vi "SDCP SMF Receiver and Transmitter - Notifiers and Queues FGV.vi"(2 "error in (no error)":errorcluster, 3 "Command":enum16{"Initialize", "Read", "Deinitialize"}(ring)) -> (0 "error out":errorcluster, 1 "Output":T1)   [LabVIEW 2020]
uses:
  Typedefs/SDCP SMF Receiver and Transmitter - Notifier and Queues.ctl
  Typedefs/SDCP SMF logger - SMF with timestamp.ctl
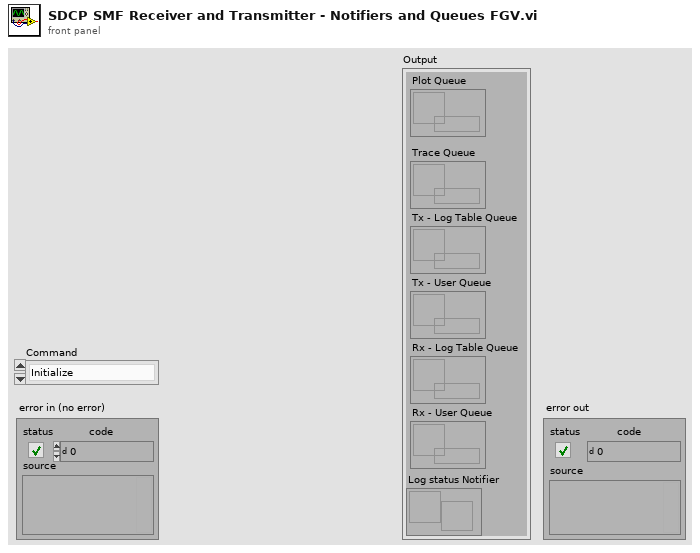
[diagram p1: front panel]
types:
  T1 = typedef "SDCP SMF Receiver and Transmitter - Notifier and Queues.ctl" = cluster{"Trace Queue":refnum<queue>, "Tx - Log Table Queue":refnum<queue>, "Tx - User Queue":refnum<queue>, "Rx - Log Table Queue":refnum<queue>, "Rx - User Queue":refnum<queue>, "Log status Notifier":refnum<notifier>, "Plot Queue":refnum<queue>}
  T2 = typedef "SDCP SMF logger - SMF with timestamp.ctl" = cluster{"Bytes":u8[], "Checksum":bool, "Time (ms)":u32, "Tx/Rx":string}
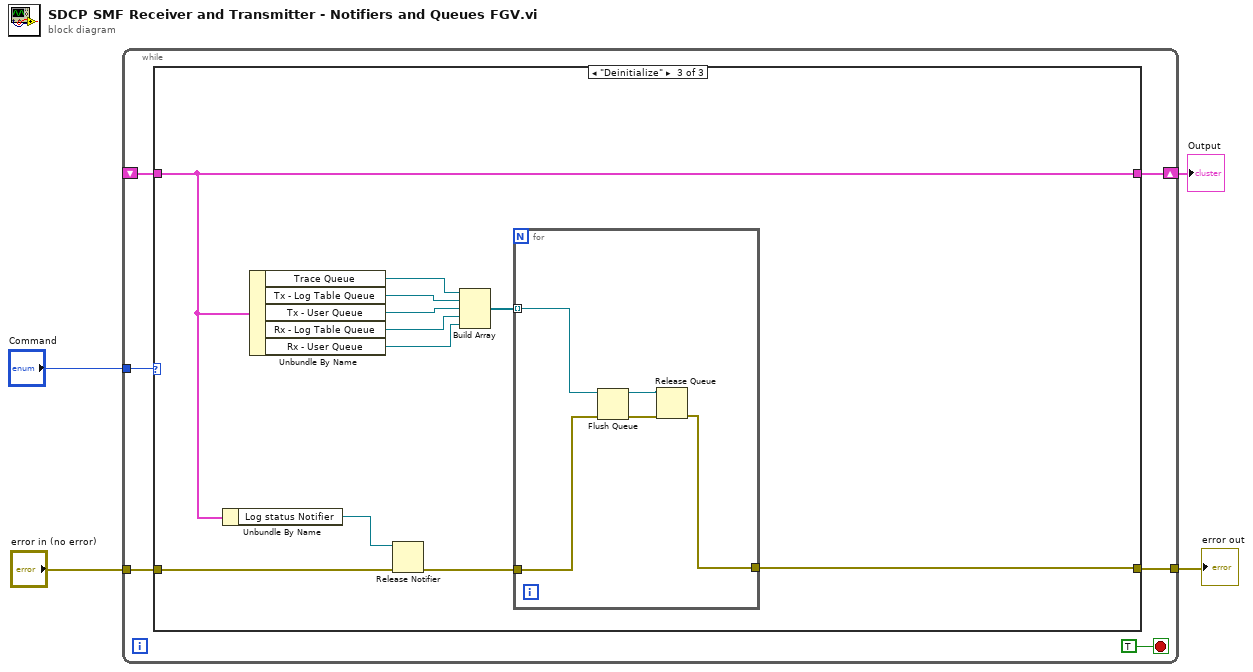
[diagram p0: block diagram]
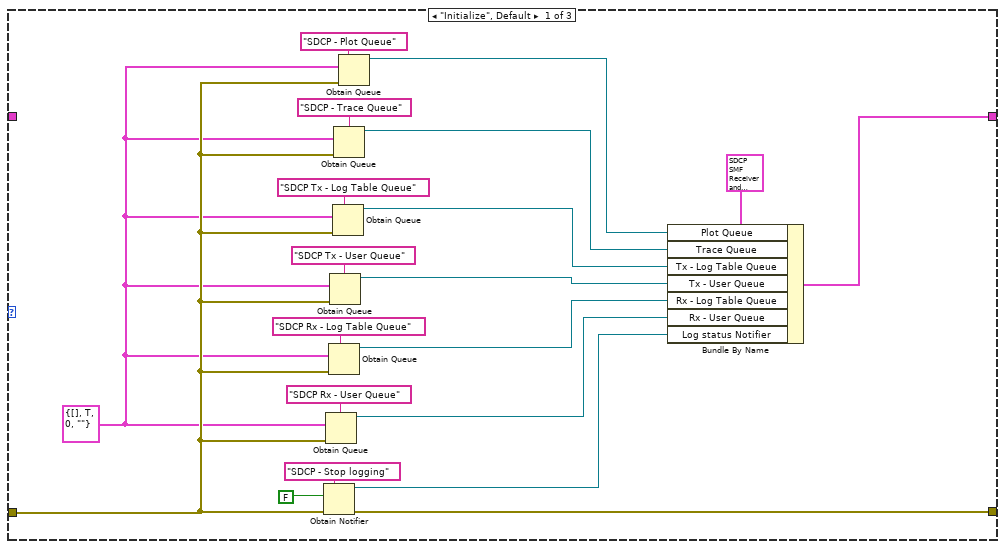
[diagram p2: hidden frame]
diagram:
  n1 = while {
    tunnel: "error in (no error)" -> [w8]
    tunnel: "Command" -> [w9]
    shift-right: [w7] -> w1
    shift-left: _ -> [w5]
    tunnel: [w6] -> w2
    stop <- TRUE stop-if-true
    n2 = case shown="\"Deinitialize\"" w9 {
      tunnel: w8 -> [w14 w31 w36]
      tunnel: [w16 w32 w37] -> w7
      tunnel: [w15 w31 w33] -> w6
      tunnel: w5 -> [_ w32 w37]
      frame "Initialize", Default {
        w13 = T2 {"Bytes"=[], "Checksum"=TRUE, "Time (ms)"=0, "Tx/Rx"=""} ("SMF with timestamp")
        n3 = Obtain Notifier(name (unnamed)="SDCP - Stop logging", notification data type=FALSE, error in (no error)=w14) -> (notifier out=w17:refnum<notifier>, error out=w15:errorcluster)  [unwired: 1 in, 1 out]
        n4 = Obtain Queue(name (unnamed)="SDCP Rx - User Queue", element data type=w13, error in (no error)=w14) -> (queue out=w18:refnum<queue>)  [unwired: 2 in, 2 out]
        n5 = Obtain Queue(name (unnamed)="SDCP Rx - Log Table Queue", element data type=w13, error in (no error)=w14) -> (queue out=w19:refnum<queue>)  [unwired: 2 in, 2 out]
        n6 = Obtain Queue(name (unnamed)="SDCP Tx - User Queue", element data type=w13, error in (no error)=w14) -> (queue out=w20:refnum<queue>)  [unwired: 2 in, 2 out]
        n7 = Obtain Queue(name (unnamed)="SDCP Tx - Log Table Queue", element data type=w13, error in (no error)=w14) -> (queue out=w21:refnum<queue>)  [unwired: 2 in, 2 out]
        n8 = Obtain Queue(name (unnamed)="SDCP - Trace Queue", element data type=w13, error in (no error)=w14) -> (queue out=w22:refnum<queue>)  [unwired: 2 in, 2 out]
        n9 = Obtain Queue(name (unnamed)="SDCP - Plot Queue", element data type=w13, error in (no error)=w14) -> (queue out=w11:refnum<queue>)  [unwired: 2 in, 2 out]
        n10 = Bundle By Name(cluster=T1 {"Trace Queue"=refnum, "Tx - Log Table Queue"=refnum, "Tx - User Queue"=refnum, "Rx - Log Table Queue"=refnum, "Rx - User Queue"=refnum, "Log status Notifier"=refnum, "Plot Queue"=refnum}, "Plot Queue"=w11, "Trace Queue"=w22, "Tx - Log Table Queue"=w21, "Tx - User Queue"=w20, "Rx - Log Table Queue"=w19, "Rx - User Queue"=w18, "Log status Notifier"=w17) -> (w16:T1)
      }
      frame "Read" {
      }
      frame "Deinitialize" {
        n11 = Unbundle By Name(w37) -> ("Log status Notifier"=w35:refnum<notifier>)
        n12 = Unbundle By Name(w37) -> ("Trace Queue"=w43:refnum<queue>, "Tx - Log Table Queue"=w42:refnum<queue>, "Tx - User Queue"=w41:refnum<queue>, "Rx - Log Table Queue"=w40:refnum<queue>, "Rx - User Queue"=w39:refnum<queue>)
        n13 = Release Notifier(notifier=w35, error in (no error)=w36) -> (error out=w34:errorcluster)  [unwired: 1 in, 2 out]
        n14 = Build Array(w43, w42, w41, w40, w39) -> (w38:refnum<queue>[])
        n15 = for {
          tunnel: w38 -> [w46] mode=indexing
          tunnel: w34 -> [w47]
          tunnel: [w48] -> w33
          n16 = Flush Queue(queue=w46, error in (no error)=w47) -> (queue out=w45:refnum<queue>, error out=w44:errorcluster)  [unwired: 1 out]
          n17 = Release Queue(queue=w45, error in (no error)=w44) -> (error out=w48:errorcluster)  [unwired: 1 in, 2 out]
        }
      }
    }
  }
  "error out" <- w2
  "Output" <- w1
